vi "PatternGen.vi"(0 "U_timing":cluster{"ON":u32, "OFF":u32}, 1 "Period":u32, 2 "Deadtime":u8=1, 5 "V_timing":cluster{"ON":u32, "OFF":u32}, 7 "W_timing":cluster{"ON":u32, "OFF":u32}, 11 "enable":bool=TRUE) -> (4 "SwitchPositions":T1)   [LabVIEW 2015, in "SVPWM.lvlib"]
uses:
  SVPWM.lvlib
  SwitchPositions.ctl
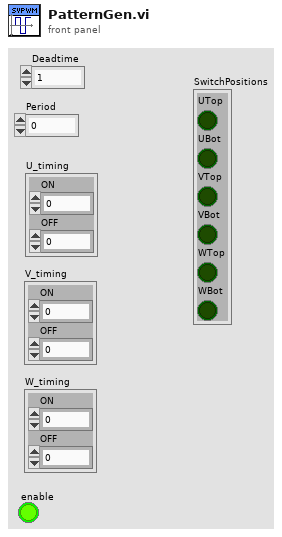
[diagram p1: front panel]
types:
  T1 = typedef "SVPWM.lvlib/SwitchPositions.ctl" = cluster{"UTop":bool, "UBot":bool, "VTop":bool, "VBot":bool, "WTop":bool, "WBot":bool}
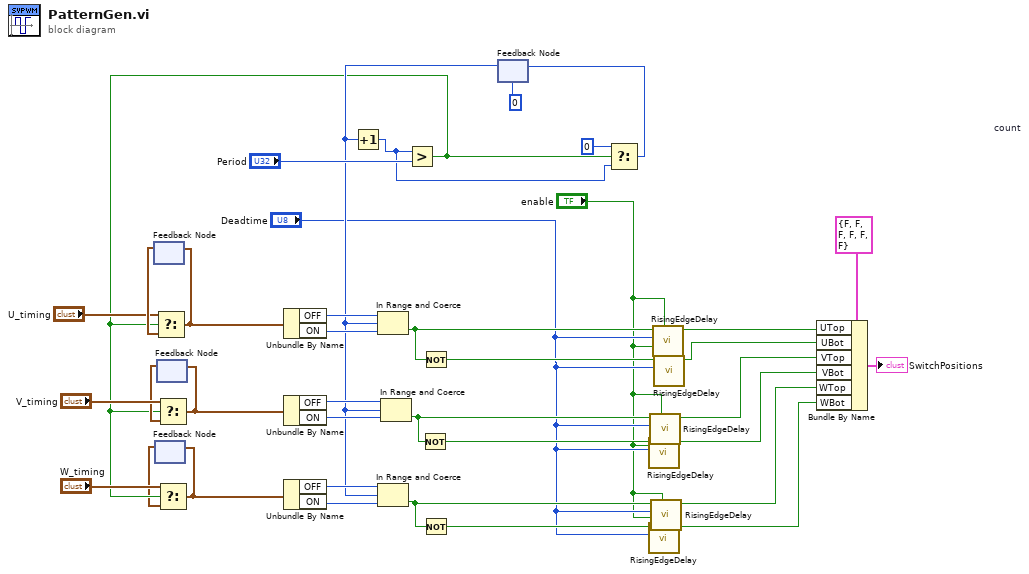
[diagram p0: block diagram]
diagram:
  n1 = feedback #1() -> (w10:cluster{"ON":u32, "OFF":u32})  [unwired: 1 in]
  n2 = feedback #2() -> (w3:cluster{"ON":u32, "OFF":u32})  [unwired: 1 in]
  n3 = feedback #3() -> (w7:cluster{"ON":u32, "OFF":u32})  [unwired: 1 in]
  n4 = feedback #4 "count"(u32 0 ("Period")) -> (w23:u32)
  n5 = Increment(x=w23) -> (x+1=w36:u32)
  n6 = Greater?(x=w36, y="Period") -> (0:w4:bool)
  n7 = Select(t="U_timing", s=w4, f=w10) -> (s? t:f=w1:cluster{"ON":u32, "OFF":u32})
  n8 = feedback-in #1(w1) -> ()
  n9 = Select(t="V_timing", s=w4, f=w7) -> (s? t:f=w6:cluster{"ON":u32, "OFF":u32})
  n10 = feedback-in #3(w6) -> ()
  n11 = Select(t="W_timing", s=w4, f=w3) -> (s? t:f=w2:cluster{"ON":u32, "OFF":u32})
  n12 = feedback-in #2(w2) -> ()
  n13 = Unbundle By Name(w1) -> ("OFF"=w33:u32, "ON"=w32:u32)
  n14 = Unbundle By Name(w6) -> ("OFF"=w28:u32, "ON"=w29:u32)
  n15 = Unbundle By Name(w2) -> ("OFF"=w25:u32, "ON"=w24:u32)
  n16 = In Range and Coerce(upper limit=w33, x=w23, lower limit=w32) -> (In Range?=w30:bool)  [unwired: 1 out]
  n17 = In Range and Coerce(upper limit=w25, x=w23, lower limit=w24) -> (In Range?=w22:bool)  [unwired: 1 out]
  n18 = In Range and Coerce(upper limit=w28, x=w23, lower limit=w29) -> (In Range?=w26:bool)  [unwired: 1 out]
  n19 = Not(x=w26) -> (.not. x?=w27:bool)
  n20 = Not(x=w30) -> (.not. x?=w31:bool)
  n21 = Not(x=w22) -> (.not. x?=w21:bool)
  n22 = Select(t=u32 0, s=w4, f=w36) -> (s? t:f=w34:u32)
  n23 = feedback-in #4(w34) -> ()
  n24 = call "RisingEdgeDelay.vi"("enable?"="enable", "Deadtime (iterations)"="Deadtime", "Input"=w27) -> ("Output"=w14:bool)  [unwired: 8 in]
  n25 = call "RisingEdgeDelay.vi"("enable?"="enable", "Deadtime (iterations)"="Deadtime", "Input"=w21) -> ("Output"=w12:bool)  [unwired: 8 in]
  n26 = call "RisingEdgeDelay.vi"("enable?"="enable", "Deadtime (iterations)"="Deadtime", "Input"=w26) -> ("Output"=w15:bool)  [unwired: 8 in]
  n27 = call "RisingEdgeDelay.vi"("enable?"="enable", "Deadtime (iterations)"="Deadtime", "Input"=w22) -> ("Output"=w13:bool)  [unwired: 8 in]
  n28 = call "RisingEdgeDelay.vi"("enable?"="enable", "Deadtime (iterations)"="Deadtime", "Input"=w30) -> ("Output"=w17:bool)  [unwired: 8 in]
  n29 = call "RisingEdgeDelay.vi"("enable?"="enable", "Deadtime (iterations)"="Deadtime", "Input"=w31) -> ("Output"=w16:bool)  [unwired: 8 in]
  n30 = Bundle By Name(cluster=T1 {"UTop"=FALSE, "UBot"=FALSE, "VTop"=FALSE, "VBot"=FALSE, "WTop"=FALSE, "WBot"=FALSE} ("SwitchPositions"), "UTop"=w17, "UBot"=w16, "VTop"=w15, "VBot"=w14, "WTop"=w13, "WBot"=w12) -> (→"SwitchPositions":T1)
